vi "OFDM_SymbolMaping.vi"(8 "error in (no error)":errorcluster, 10 "Modulation type":T1(ring), 11 "input bit stream":i8[](array[numeric])) -> (0 "error out":errorcluster, 3 "symbols":cdb[](array[numeric]))   [LabVIEW 2022 SP3]
uses:
  <vilib>/addons/Modulation/Digital/General/MT Map Bits to QAM Symbols.vi
  <vilib>/addons/Modulation/Digital/General/MT Map Bits to PSK Symbols.vi
  <vilib>/addons/Modulation/niDMT.lvlib
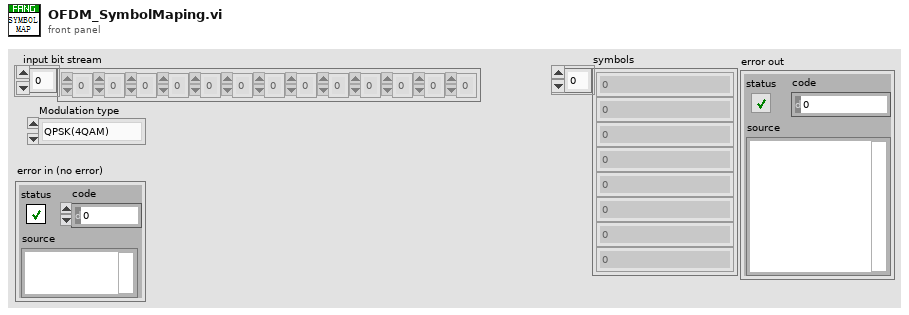
[diagram p1: front panel]
types:
  T1 = enum16{"QPSK(4QAM)", "64QAM", "16QAM", "BPSK", "BPSK Vertical"}
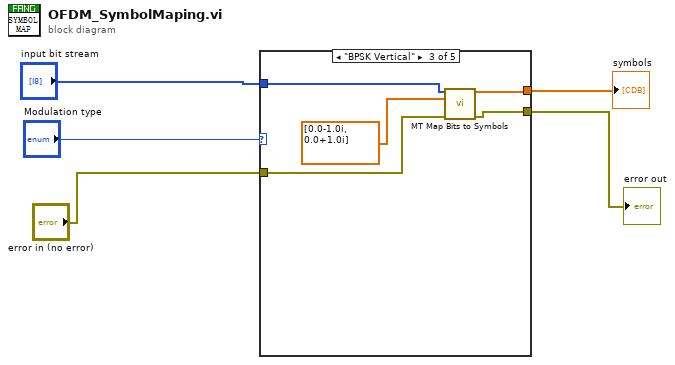
[diagram p0: block diagram]
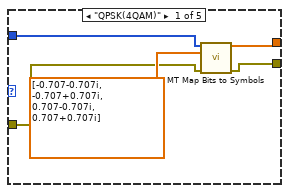
[diagram p2: hidden frame]
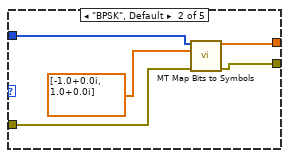
[diagram p3: hidden frame]
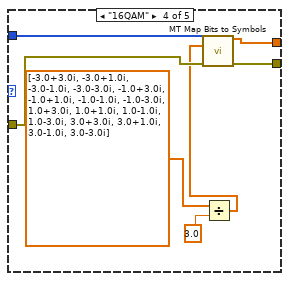
[diagram p4: hidden frame]
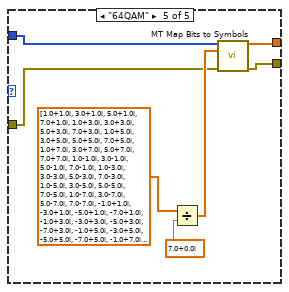
[diagram p5: hidden frame]
diagram:
  n1 = case shown="\"BPSK Vertical\"" "Modulation type" {
    tunnel: [w10 w11 w19 w25 w28] -> w2
    tunnel: "error in (no error)" -> [w7 w13 w17 w27 w30]
    tunnel: "input bit stream" -> [w9 w15 w16 w26 w31]
    tunnel: [w6 w12 w18 w24 w29] -> w1
    frame "QPSK(4QAM)" {
      n2 = call-poly <vilib>:"MT Map Bits to Symbols.vi"("input bit stream"=w9, "symbol map"=cdb[] [-0.707-0.707i, -0.707+0.707i, 0.707-0.707i, 0.707+0.707i], "error in (no error)"=w7) -> ("symbols"=w10:cdb[], "error out"=w6:errorcluster)  [unwired: 11 in]
    }
    frame "BPSK", Default {
      n3 = call-poly <vilib>:"MT Map Bits to Symbols.vi"("input bit stream"=w15, "symbol map"=cdb[] [-1.0+0.0i, 1.0+0.0i], "error in (no error)"=w13) -> ("symbols"=w11:cdb[], "error out"=w12:errorcluster)  [unwired: 11 in]
    }
    frame "BPSK Vertical" {
      n4 = call-poly <vilib>:"MT Map Bits to Symbols.vi"("input bit stream"=w16, "symbol map"=cdb[] [0.0-1.0i, 0.0+1.0i], "error in (no error)"=w17) -> ("symbols"=w19:cdb[], "error out"=w18:errorcluster)  [unwired: 11 in]
    }
    frame "16QAM" {
      n5 = Divide(x=cdb[] [-3.0+3.0i, -3.0+1.0i, -3.0-1.0i, -3.0-3.0i, -1.0+3.0i, -1.0+1.0i, -1.0-1.0i, -1.0-3.0i, 1.0+3.0i, 1.0+1.0i, 1.0-1.0i, 1.0-3.0i, 3.0+3.0i, 3.0+1.0i, 3.0-1.0i, 3.0-3.0i] ("symbol map"), y=3.0) -> (x/y=w21:cdb[])
      n6 = call-poly <vilib>:"MT Map Bits to Symbols.vi"("input bit stream"=w26, "symbol map"=w21, "error in (no error)"=w27) -> ("symbols"=w25:cdb[], "error out"=w24:errorcluster)  [unwired: 11 in]
    }
    frame "64QAM" {
      n7 = Divide(x=cdb[] [1.0+1.0i, 3.0+1.0i, 5.0+1.0i, 7.0+1.0i, 1.0+3.0i, 3.0+3.0i, 5.0+3.0i, 7.0+3.0i, 1.0+5.0i, 3.0+5.0i, 5.0+5.0i, 7.0+5.0i, 1.0+7.0i, 3.0+7.0i, 5.0+7.0i, 7.0+7.0i, 1.0-1.0i, 3.0-1.0i, 5.0-1.0i, 7.0-1.0i, 1.0-3.0i, 3.0-3.0i, 5.0-3.0i, 7.0-3.0i, 1.0-5.0i, 3.0-5.0i, 5.0-5.0i, 7.0-5.0i, 1.0-7.0i, 3.0-7.0i, 5.0-7.0i, 7.0-7.0i, -1.0+1.0i, -3.0+1.0i, -5.0+1.0i, -7.0+1.0i, -1.0+3.0i, -3.0+3.0i, -5.0+3.0i, -7.0+3.0i, -1.0+5.0i, -3.0+5.0i, -5.0+5.0i, -7.0+5.0i, -1.0+7.0i, -3.0+7.0i, -5.0+7.0i, -7.0+7.0i, -1.0-1.0i, -3.0-1.0i, -5.0-1.0i, -7.0-1.0i, -1.0-3.0i, -3.0-3.0i, -5.0-3.0i, -7.0-3.0i, -1.0-5.0i, -3.0-5.0i, -5.0-5.0i, -7.0-5.0i, -1.0-7.0i, -3.0-7.0i, -5.0-7.0i, -7.0-7.0i] ("appended array"), y=cdb 7.0+0.0i) -> (x/y=w33:cdb[])
      n8 = call-poly <vilib>:"MT Map Bits to Symbols.vi"("input bit stream"=w31, "symbol map"=w33, "error in (no error)"=w30) -> ("symbols"=w28:cdb[], "error out"=w29:errorcluster)  [unwired: 11 in]
    }
  }
  "symbols" <- w2
  "error out" <- w1
